vi "3-2.vi"() -> ()   [LabVIEW 2017]
panel:
  out "Cluster Array":T1(array[cluster])
  in  "Array 3":bool[](array[boolean])
  in  "Array 2":dbl[](array[numeric])
  in  "Array":dbl[](array[numeric])
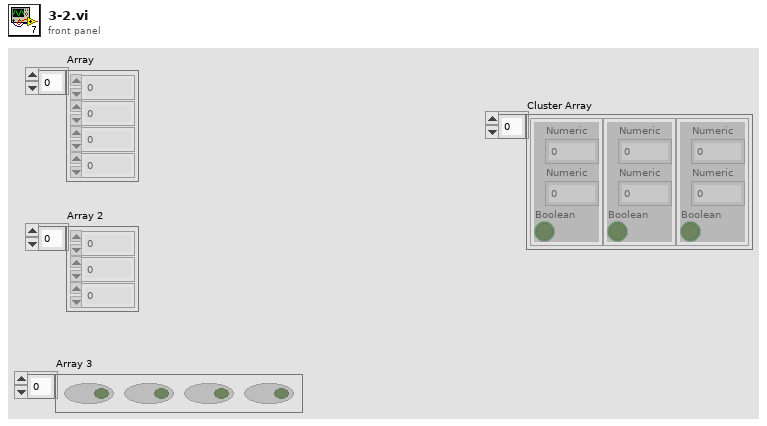
[diagram p1: front panel]
types:
  T1 = cluster{"Numeric":dbl, "Numeric":dbl, "Boolean":bool}[]
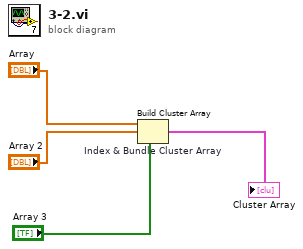
[diagram p0: block diagram]
diagram:
  n1 = Build Cluster Array "Index & Bundle Cluster Array"("Array", "Array 2", "Array 3") -> (→"Cluster Array":T1)
